vi "input_fifos.vi"(11 "Offline size":i32=150) -> (0 "error out":errorcluster, 2 "queue out 2":refnum<queue>, 3 "Queue out":refnum<queue>)   [LabVIEW 2026]
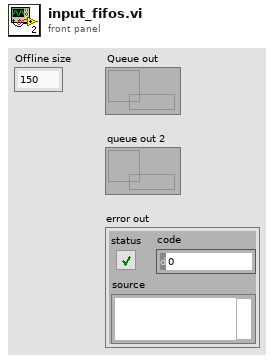
[diagram p1: front panel]
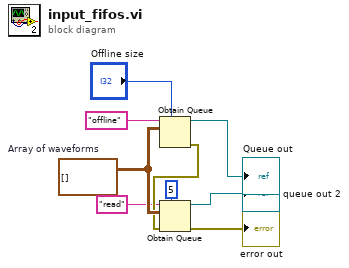
[diagram p0: block diagram]
diagram:
  w7 = waveform(dbl)[][] []  # Array of waveforms
  n1 = Obtain Queue(max queue size (-1, unlimited)="Offline size", name (unnamed)="offline", element data type=w7) -> (queue out=→"Queue out":refnum<queue>, error out=w5:errorcluster)  [unwired: 2 in, 1 out]
  n2 = Obtain Queue(max queue size (-1, unlimited)=5, name (unnamed)="read", element data type=w7, error in (no error)=w5) -> (queue out=→"queue out 2":refnum<queue>, error out=→"error out":errorcluster)  [unwired: 1 in, 1 out]
